vi "buntopenning.vi"() -> ()   [LabVIEW 2014, in "Panels.lvlib"]
uses:
  Panels.lvlib
  CSlibraries-extern/DimLVEvent/DimIndicators/DimIndicators.lvlib
  CSlibraries/UtilityLib/UtilityLib.lvlib
  CS_Core/CSSystem/CoreLib/CoreLib.lvlib
  CSlibraries/UtilityLib/UtilityLib.valueStatus.ctl
  CSlibraries-extern/DimLVEvent/LVDimInterface/LVDimInterface.lvlib
  Instance           1 20Saved   BuntoPenning .vi
  CSlibraries-extern/DimLVEvent/DimIndicators/DimIndicators.numericType.ctl
  CSlibraries-extern/DimLVEvent/DimIndicators/DimIndicators.numericArrayType.ctl
  CSlibraries-extern/DimLVEvent/DimIndicators/DimIndicators.anyType.ctl
panel:
  in  "SetFileLocation_Data":T1={"data"="NOLINK", "no link"=TRUE, "quality"=-1, "timeStamp"=0.0}
  in  "InjPenC":bool
  in  "InjPenB":bool
  in  "InjPenA":bool
  in  "InjPenBaseY":bool
  in  "InjPenBaseX":bool
  in  "InjPenDTBase1":bool
  in  "ELens8":bool
  in  "BOB5DefY":bool
  in  "BOB5DefX":bool
  in  "BOB4DefY":bool
  in  "BOB4DefX":bool
  in  "ELens7":bool
  in  "ELens6":bool
  in  "PulsedDT1":bool
  in  "PulsedDT2":bool
  in  "ELens8_SetData":T2={"data"=[0.0, 0.0, 0.0, 0.0], "no link"=FALSE, "quality"=0, "timeStamp"=3268667320.388}
  in  "SetFileLocation":path=path "\\\\intranet\\Files/projects/lebit/Data Exchange/data/buntopenningControl"
  in  "PulsedDT1_SetValueInfoData":T2={"data"=[-120.0, 120.0, -1.0], "no link"=FALSE, "quality"=0, "timeStamp"=3268667320.404}
  in  "PulsedDT1_SetData":T2={"data"=[0.0, 0.0, 0.0, 0.0], "no link"=FALSE, "quality"=0, "timeStamp"=3268667320.388}
  in  "PulsedDT1_MonData":T3={"data"=inf, "no link"=FALSE, "quality"=1, "timeStamp"=3268667320.373}
  in  "BOB4DefY_MonData":T3={"data"=inf, "no link"=FALSE, "quality"=1, "timeStamp"=3268667320.373}
  in  "ELens7_MonData":T3={"data"=inf, "no link"=FALSE, "quality"=1, "timeStamp"=3268667320.373}
  in  "BOB5DefX_MonData":T3={"data"=inf, "no link"=FALSE, "quality"=1, "timeStamp"=3268667320.373}
  in  "BOB5DefY_MonData":T3={"data"=inf, "no link"=FALSE, "quality"=1, "timeStamp"=3268667320.373}
  in  "ELens8_MonData":T3={"data"=inf, "no link"=TRUE, "quality"=-1, "timeStamp"=0.0}
  in  "InjPenDTBase1_MonData":T3={"data"=inf, "no link"=FALSE, "quality"=1, "timeStamp"=3268667320.373}
  in  "BOB4DefX_MonData":T3={"data"=inf, "no link"=FALSE, "quality"=1, "timeStamp"=3268667320.373}
  in  "ELens6_MonData":T3={"data"=inf, "no link"=FALSE, "quality"=1, "timeStamp"=3268667320.373}
  in  "BOB4Keithley_MonData":T3={"data"=inf, "no link"=FALSE, "quality"=1, "timeStamp"=3268667320.373}
  in  "PulsedDT2_MonData":T3={"data"=inf, "no link"=TRUE, "quality"=-1, "timeStamp"=0.0}
  in  "InjPenBaseY_MonData":T3={"data"=inf, "no link"=TRUE, "quality"=-1, "timeStamp"=0.0}
  in  "InjPenB_MonData":T3={"data"=inf, "no link"=FALSE, "quality"=1, "timeStamp"=3268667320.388}
  in  "InjPenBaseX_MonData":T3={"data"=inf, "no link"=TRUE, "quality"=-1, "timeStamp"=0.0}
  in  "InjPenA_MonData":T3={"data"=inf, "no link"=FALSE, "quality"=1, "timeStamp"=3268667320.388}
  in  "InjPenC_MonData":T3={"data"=inf, "no link"=FALSE, "quality"=1, "timeStamp"=3268667320.388}
  out "PulsedDT2_Mon":dbl=inf format="%.4f"
  out "InjPenC_Mon":dbl=inf format="%.4f"
  out "InjPenB_Mon":dbl=inf format="%.4f"
  out "InjPenA_Mon":dbl=inf format="%.4f"
  in  "PulsedDT2_SetValueInfoData":T2={"data"=[], "no link"=TRUE, "quality"=-1, "timeStamp"=0.0}
  in  "PulsedDT2_SetData":T2={"data"=[], "no link"=TRUE, "quality"=-1, "timeStamp"=0.0}
  in  "InjPenC_SetValueInfoData":T2={"data"=[0.0, 1500.0, -1.0], "no link"=FALSE, "quality"=0, "timeStamp"=3268667320.42}
  in  "InjPenBaseY_SetValueInfoData":T2={"data"=[], "no link"=TRUE, "quality"=-1, "timeStamp"=0.0}
  in  "InjPenBaseX_SetValueInfoData":T2={"data"=[], "no link"=TRUE, "quality"=-1, "timeStamp"=0.0}
  in  "InjPenB_SetValueInfoData":T2={"data"=[-400.0, 400.0, -1.0], "no link"=FALSE, "quality"=0, "timeStamp"=3268667320.42}
  in  "InjPenA_SetValueInfoData":T2={"data"=[-400.0, 400.0, -1.0], "no link"=FALSE, "quality"=0, "timeStamp"=3268667320.42}
  in  "InjPenC_SetData":T2={"data"=[0.0, 0.0, 0.0, 0.0], "no link"=FALSE, "quality"=0, "timeStamp"=3268667320.404}
  in  "InjPenBaseY_SetData":T2={"data"=[], "no link"=TRUE, "quality"=-1, "timeStamp"=0.0}
  in  "InjPenBaseX_SetData":T2={"data"=[], "no link"=TRUE, "quality"=-1, "timeStamp"=0.0}
  in  "InjPenB_SetData":T2={"data"=[0.0, 0.0, 0.0, 0.0], "no link"=FALSE, "quality"=0, "timeStamp"=3268667320.404}
  in  "InjPenA_SetData":T2={"data"=[0.0, 0.0, 0.0, 0.0], "no link"=FALSE, "quality"=0, "timeStamp"=3268667320.404}
  out "ELens7_Mon":dbl=inf format="%.4f"
  out "InjPenDTBase1_Mon":dbl=inf format="%.4f"
  out "ELens6_Mon":dbl=inf format="%.4f"
  out "ELens8_Mon":dbl=inf format="%.4f"
  out "InjPenBaseX_Mon":dbl=inf format="%.4f"
  out "PulsedDT1_Mon":dbl=inf format="%.4f"
  out "i ref out":refnum<vi>
  in  "Last Loaded File_Data":T1={"data"="NOLINK", "no link"=TRUE, "quality"=-1, "timeStamp"=0.0}
  out "FileUpToDate":bool=TRUE caption="Parameter Changed"
  in  "Close All Panels":bool
  in  "BOB4DefX_SetValueInfoData":T2={"data"=[], "no link"=TRUE, "quality"=-1, "timeStamp"=0.0}
  in  "BOB4DefY_SetValueInfoData":T2={"data"=[-400.0, 400.0, -1.0], "no link"=FALSE, "quality"=0, "timeStamp"=3268667320.42}
  in  "ELens7_SetValueInfoData":T2={"data"=[0.0, 5000.0, -1.0], "no link"=FALSE, "quality"=0, "timeStamp"=3268667320.42}
  in  "BOB5DefX_SetValueInfoData":T2={"data"=[-400.0, 400.0, -1.0], "no link"=FALSE, "quality"=0, "timeStamp"=3268667320.42}
  in  "BOB5DefY_SetValueInfoData":T2={"data"=[-400.0, 400.0, -1.0], "no link"=FALSE, "quality"=0, "timeStamp"=3268667320.42}
  in  "ELens8_SetValueInfoData":T2={"data"=[], "no link"=TRUE, "quality"=-1, "timeStamp"=0.0}
  in  "InjPenDTBase1_SetValueInfoData":T2={"data"=[0.0, 3000.0, -1.0], "no link"=FALSE, "quality"=0, "timeStamp"=3268667320.42}
  in  "ELens6_SetValueInfoData":T2={"data"=[0.0, 5000.0, -1.0], "no link"=FALSE, "quality"=0, "timeStamp"=3268667320.404}
  in  "InjPenDTBase1_SetData":T2={"data"=[0.0, 0.0, 0.0, 0.0], "no link"=FALSE, "quality"=0, "timeStamp"=3268667320.388}
  in  "BOB5DefY_SetData":T2={"data"=[0.0, 0.0, 0.0, 0.0], "no link"=FALSE, "quality"=0, "timeStamp"=3268667320.388}
  in  "BOB5DefX_SetData":T2={"data"=[0.0, 0.0, 0.0, 0.0], "no link"=FALSE, "quality"=0, "timeStamp"=3268667320.388}
  in  "ELens7_SetData":T2={"data"=[0.0, 0.0, 0.0, 0.0], "no link"=FALSE, "quality"=0, "timeStamp"=3268667320.388}
  in  "BOB4DefY_SetData":T2={"data"=[0.0, 0.0, 0.0, 0.0], "no link"=FALSE, "quality"=0, "timeStamp"=3268667320.388}
  in  "BOB4DefX_SetData":T2={"data"=[0.0, 0.0, 0.0, 0.0], "no link"=FALSE, "quality"=0, "timeStamp"=3268667320.388}
  in  "ELens6_SetData":T2={"data"=[0.0, 0.0, 0.0, 0.0], "no link"=FALSE, "quality"=0, "timeStamp"=3268667320.388}
  out "Last Loaded File":string
  out "BOB5DefY_Mon":dbl=inf format="%.4f"
  out "InjPenBaseY_Mon":dbl=inf format="%.4f"
  out "BOB4DefY_Mon":dbl=inf format="%.4f"
  out "BOB5DefX_Mon":dbl=inf format="%.4f"
  out "BOB4DefX_Mon":dbl=inf format="%.4f"
  # "Parameter changed, data file is no longer up-to-date."
  # "Values in italic don't have a real monitor"
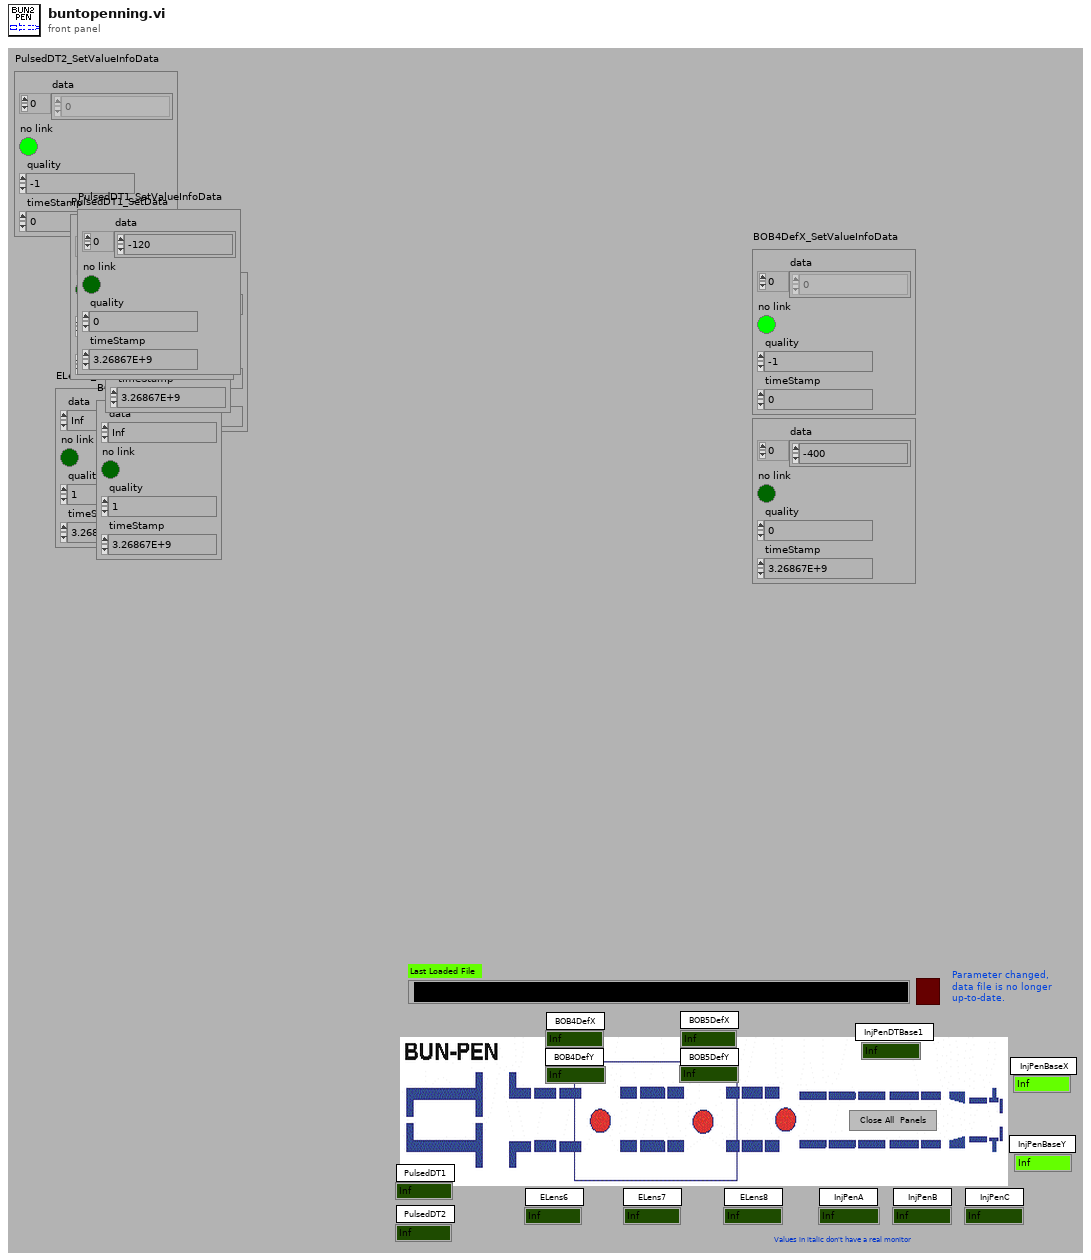
[diagram p1: front panel]
types:
  T1 = typedef "DimIndicators.lvlib/DimIndicators.anyType.ctl" = cluster{"data":string, "no link":bool, "quality":i32, "timeStamp":dbl}
  T2 = typedef "DimIndicators.lvlib/DimIndicators.numericArrayType.ctl" = cluster{"data":dbl[], "no link":bool, "quality":i32, "timeStamp":dbl}
  T3 = typedef "DimIndicators.lvlib/DimIndicators.numericType.ctl" = cluster{"data":dbl, "no link":bool, "quality":i32, "timeStamp":dbl}
  T4 = typedef "UtilityLib.lvlib/UtilityLib.valueStatus.ctl" = enum16{"no info available", "stand by/off", "on", "warning", "alarm/malfunction", "not implemented", "user action required", "important information", "system default", "control default", "indicator default", "button default"}
  T5 = cluster{"data":string, "no link":bool, "quality":i32, "timeStamp":dbl}
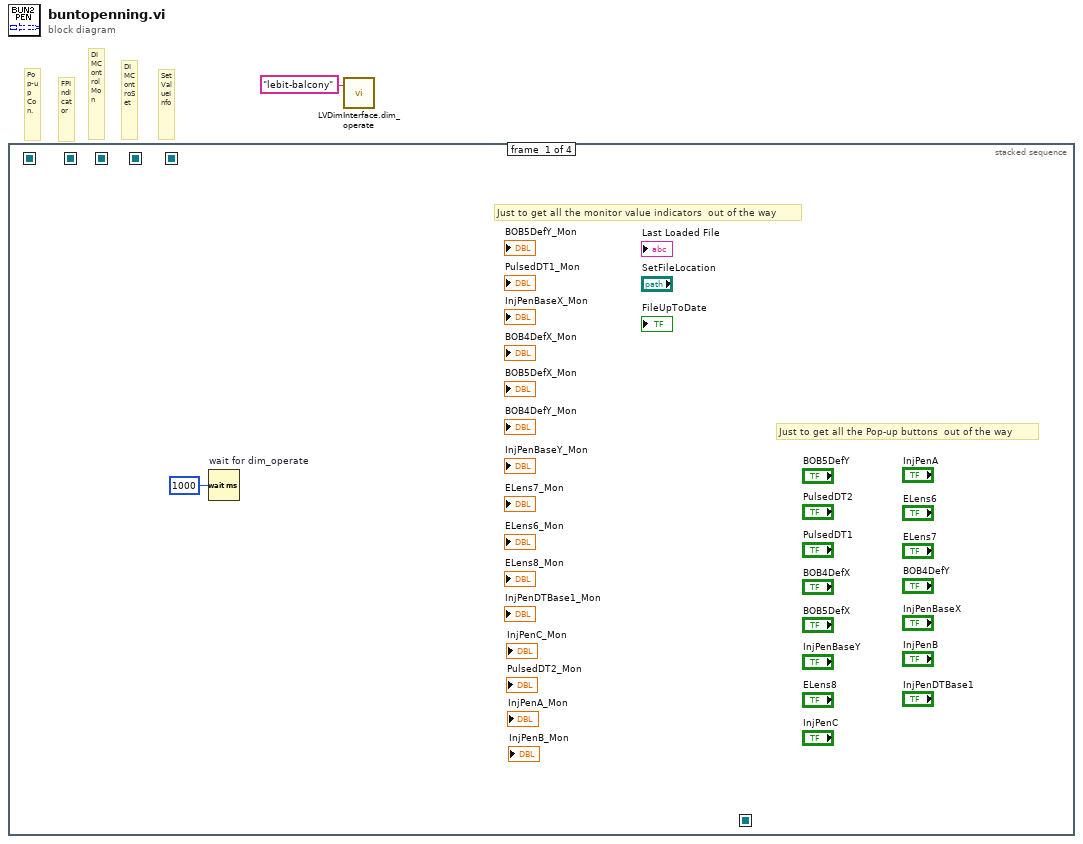
[diagram p0: block diagram]
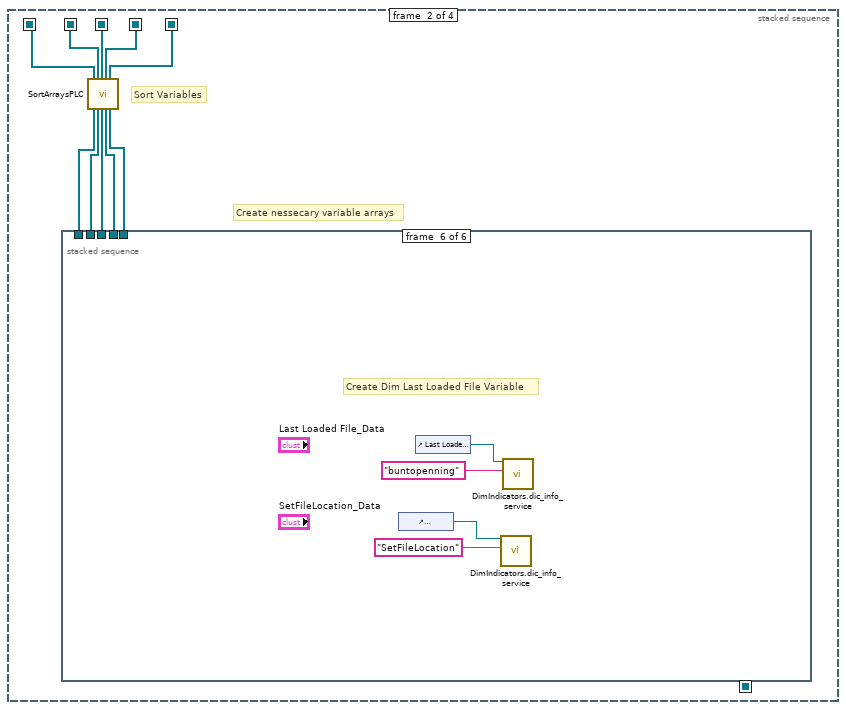
[diagram p2: hidden frame]
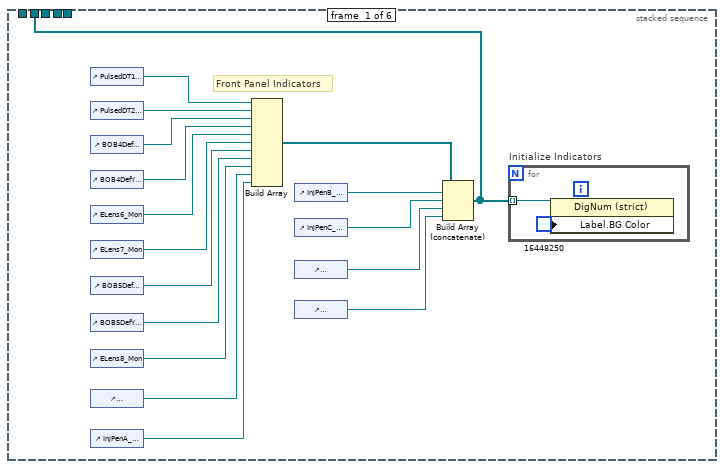
[diagram p3: hidden frame]
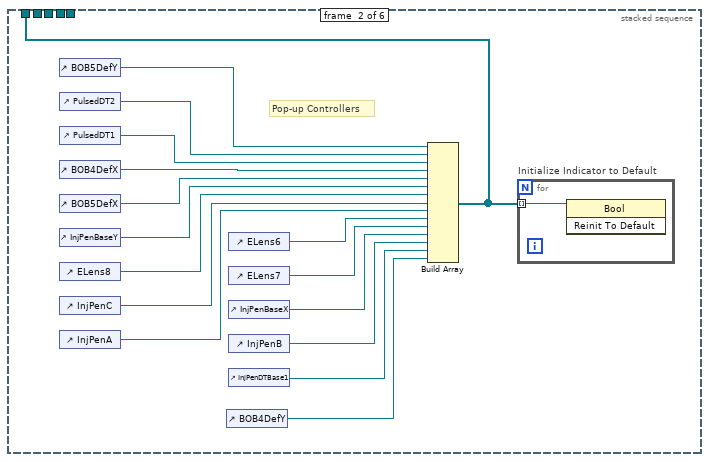
[diagram p4: hidden frame]
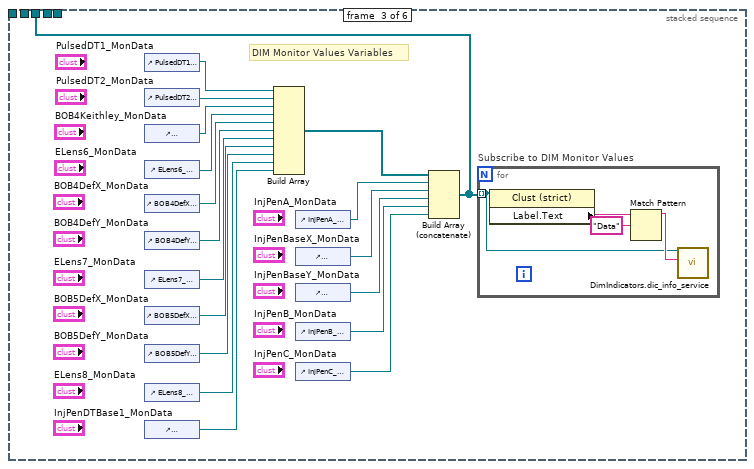
[diagram p5: hidden frame]
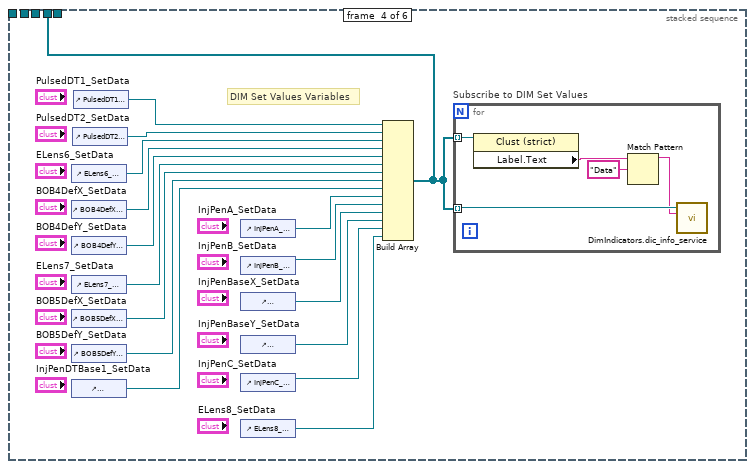
[diagram p6: hidden frame]
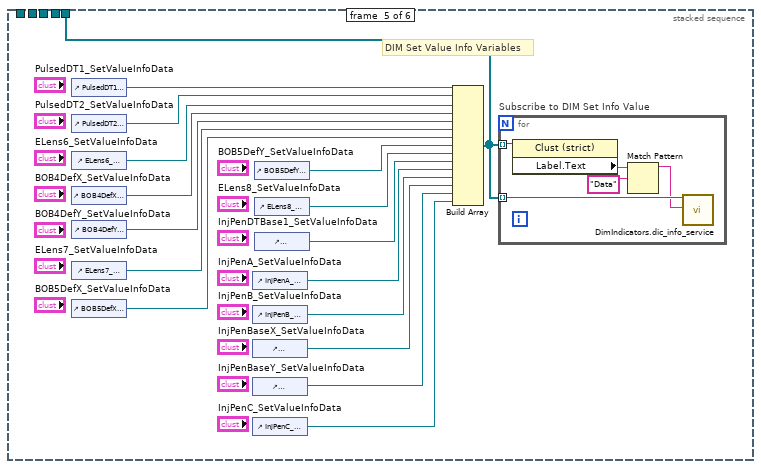
[diagram p7: hidden frame]
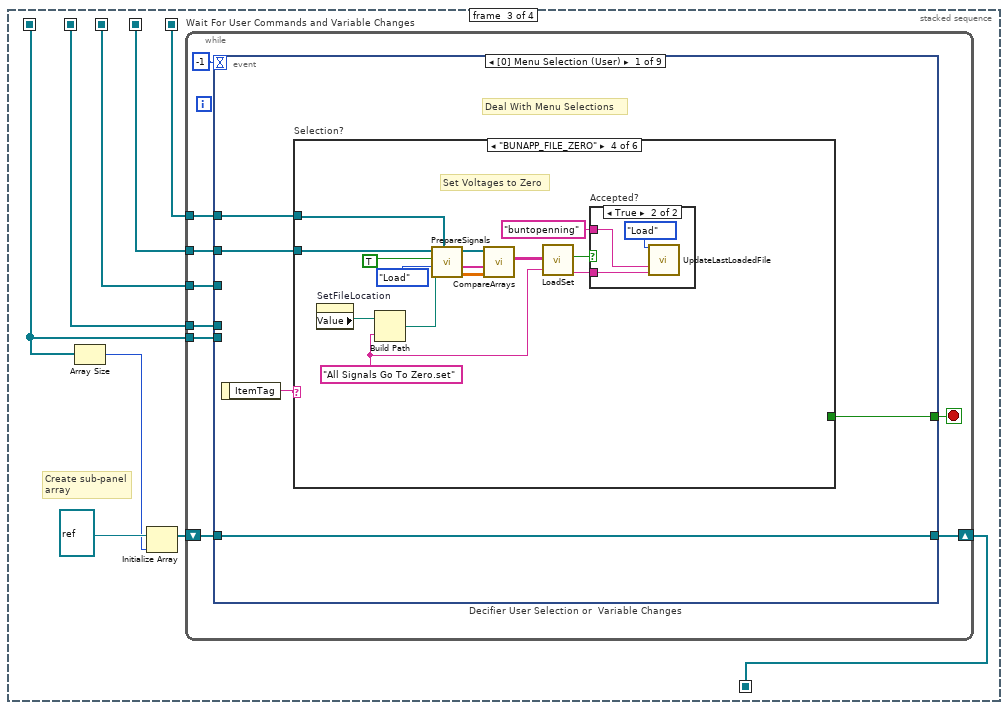
[diagram p8: hidden frame]
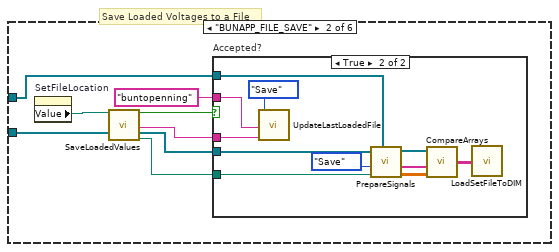
[diagram p10: hidden frame]
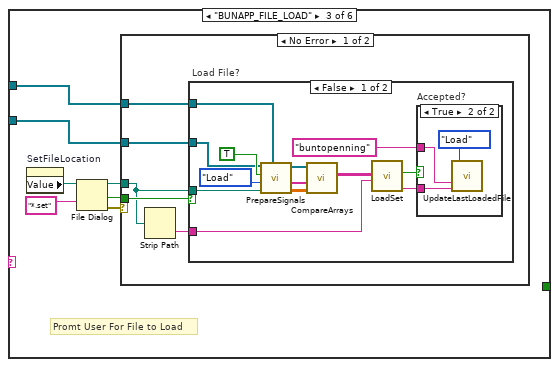
[diagram p12: hidden frame]
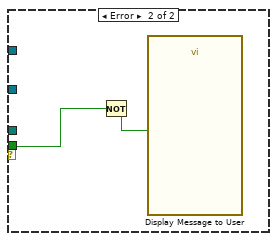
[diagram p15: hidden frame]
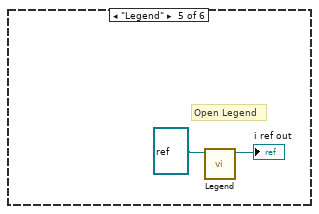
[diagram p17: hidden frame]
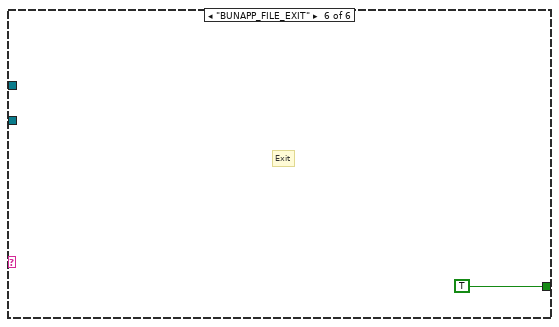
[diagram p18: hidden frame]
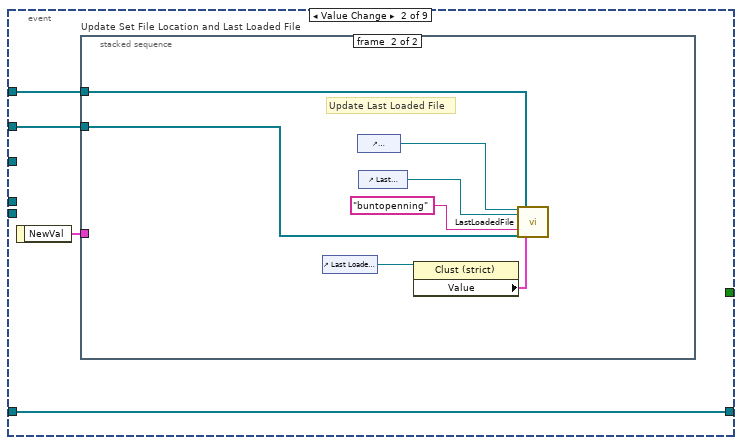
[diagram p19: hidden frame]
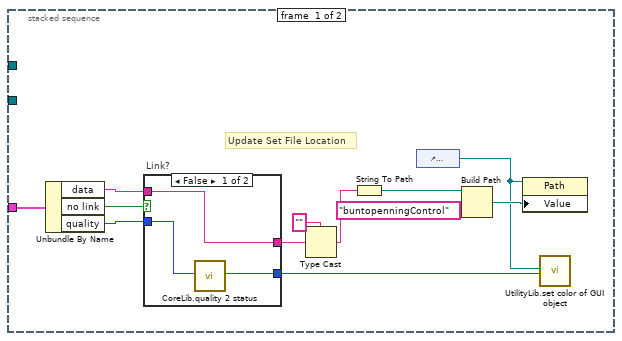
[diagram p20: hidden frame]
diagram:
  # "Pop-up Con."
  # "SetValueInfo"
  # "DIMControSet"
  # "DIMControlMon"
  # "FPIndicator"
  n1 = stacked-sequence {
    seq-local: [_ w8 _ _] -> [_ _ w119 _]
    seq-local: [_ w10 _ _] -> [_ _ w117 w318]
    seq-local: [_ _ w122 _] -> [_ _ _ w317]
    seq-local: [_ w11 _ _] -> [_ _ w121 w316]
    seq-local: [_ w12 _ _] -> [_ _ w118 w315]
    seq-local: [_ w9 _ _] -> [_ _ w120 _]
    frame #0 {
      # "Just to get all the Pop-up buttons  out of the way"
      # "Just to get all the monitor value indicators  out of the way"
      n2 = Wait (ms) "wait for dim_operate"(milliseconds to wait=u32 1000) -> ()  [unwired: 1 out]
    }
    frame #1 {
      # "Create nessecary variable arrays"
      # "Sort Variables"
      n3 = stacked-sequence {
        tunnel: [w13 _ _ _ _ _] -> w7
        tunnel: [_ w32 _ _ _ _] -> w6
        tunnel: [_ _ w49 _ _ _] -> w5
        tunnel: [_ _ _ w71 _ _] -> w4
        tunnel: [_ _ _ _ w92 _] -> w3
        frame #0 {
          # "Front Panel Indicators"
          n4 = control-ref of="PulsedDT1_Mon"() -> (w29:refnum<vi>)
          n5 = control-ref of="PulsedDT2_Mon"() -> (w25:refnum<vi>)
          n6 = control-ref of="BOB4DefX_Mon"() -> (w28:refnum<vi>)
          n7 = control-ref of="BOB4DefY_Mon"() -> (w24:refnum<vi>)
          n8 = control-ref of="ELens6_Mon"() -> (w23:refnum<vi>)
          n9 = control-ref of="ELens7_Mon"() -> (w22:refnum<vi>)
          n10 = control-ref of="BOB5DefX_Mon"() -> (w21:refnum<vi>)
          n11 = control-ref of="BOB5DefY_Mon"() -> (w20:refnum<vi>)
          n12 = control-ref of="ELens8_Mon"() -> (w19:refnum<vi>)
          n13 = control-ref of="InjPenDTBase1_Mon"() -> (w18:refnum<vi>)
          n14 = control-ref of="InjPenA_Mon"() -> (w17:refnum<vi>)
          n15 = Build Array(w29, w25, w28, w24, w23, w22, w21, w20, w19, w18, w17) -> (w27:refnum<vi>[])
          n16 = control-ref of="InjPenB_Mon"() -> (w16:refnum<vi>)
          n17 = control-ref of="InjPenC_Mon"() -> (w26:refnum<vi>)
          n18 = control-ref of="InjPenBaseX_Mon"() -> (w15:refnum<vi>)
          n19 = control-ref of="InjPenBaseY_Mon"() -> (w14:refnum<vi>)
          n20 = Build Array (concatenate)(w27, w16, w26, w15, w14) -> (w13:refnum<vi>[])
          n21 = for "Initialize Indicators" {
            tunnel: w13 -> [w31] mode=indexing
            n22 = property class="DigNum (strict)"(reference=w31, "Label.BG Color"=u32 16448250 ("Color Box")) -> ()  [unwired: 1 in, 2 out]
          }
        }
        frame #1 {
          # "Pop-up Controllers"
          n23 = control-ref of="BOB5DefY"() -> (w47:refnum<vi>)
          n24 = control-ref of="PulsedDT2"() -> (w46:refnum<vi>)
          n25 = control-ref of="PulsedDT1"() -> (w45:refnum<vi>)
          n26 = control-ref of="BOB4DefX"() -> (w44:refnum<vi>)
          n27 = control-ref of="BOB5DefX"() -> (w43:refnum<vi>)
          n28 = control-ref of="InjPenBaseY"() -> (w42:refnum<vi>)
          n29 = control-ref of="ELens8"() -> (w41:refnum<vi>)
          n30 = control-ref of="InjPenC"() -> (w40:refnum<vi>)
          n31 = control-ref of="InjPenA"() -> (w39:refnum<vi>)
          n32 = control-ref of="BOB4DefY"() -> (w33:refnum<vi>)
          n33 = control-ref of="ELens6"() -> (w38:refnum<vi>)
          n34 = control-ref of="ELens7"() -> (w37:refnum<vi>)
          n35 = control-ref of="InjPenBaseX"() -> (w36:refnum<vi>)
          n36 = control-ref of="InjPenB"() -> (w35:refnum<vi>)
          n37 = control-ref of="InjPenDTBase1"() -> (w34:refnum<vi>)
          n38 = Build Array(w47, w46, w45, w44, w43, w42, w41, w40, w39, w38, w37, w36, w35, w34, w33) -> (w32:refnum<vi>[])
          n39 = for "Initialize Indicator to Default" {
            tunnel: w32 -> [w48] mode=indexing
            n40 = invoke class="Bool" method="Reinit To Default"(reference=w48) -> ()  [unwired: 2 in, 3 out]
          }
        }
        frame #2 {
          # "DIM Monitor Values Variables"
          n41 = control-ref of="PulsedDT1_MonData"() -> (w50:refnum<vi>)
          n42 = control-ref of="PulsedDT2_MonData"() -> (w51:refnum<vi>)
          n43 = control-ref of="BOB4Keithley_MonData"() -> (w56:refnum<vi>)
          n44 = control-ref of="ELens6_MonData"() -> (w60:refnum<vi>)
          n45 = control-ref of="BOB4DefX_MonData"() -> (w59:refnum<vi>)
          n46 = control-ref of="BOB4DefY_MonData"() -> (w66:refnum<vi>)
          n47 = control-ref of="ELens7_MonData"() -> (w65:refnum<vi>)
          n48 = control-ref of="BOB5DefX_MonData"() -> (w64:refnum<vi>)
          n49 = control-ref of="BOB5DefY_MonData"() -> (w63:refnum<vi>)
          n50 = control-ref of="ELens8_MonData"() -> (w62:refnum<vi>)
          n51 = control-ref of="InjPenDTBase1_MonData"() -> (w61:refnum<vi>)
          n52 = Build Array(w50, w51, w56, w60, w59, w66, w65, w64, w63, w62, w61) -> (w53:refnum<vi>[])
          n53 = control-ref of="InjPenA_MonData"() -> (w58:refnum<vi>)
          n54 = control-ref of="InjPenBaseX_MonData"() -> (w57:refnum<vi>)
          n55 = control-ref of="InjPenBaseY_MonData"() -> (w55:refnum<vi>)
          n56 = control-ref of="InjPenB_MonData"() -> (w54:refnum<vi>)
          n57 = control-ref of="InjPenC_MonData"() -> (w52:refnum<vi>)
          n58 = Build Array (concatenate)(w53, w58, w57, w55, w54, w52) -> (w49:refnum<vi>[])
          n59 = for "Subscribe to DIM Monitor Values" {
            tunnel: w49 -> [w67] mode=indexing
            n60 = property class="Clust (strict)"(reference=w67) -> ("Label.Text"=w69:string)  [unwired: 1 in, 2 out]
            n61 = Match Pattern(string=w69, regular expression="Data") -> (before substring=w68:string)  [unwired: 1 in, 3 out]
            n62 = call "DimIndicators.dic_info_service.vi"("controlRef"=w67, "serviceName"=w68) -> ()  [unwired: 16 in, 2 out]
          }
        }
        frame #3 {
          # "DIM Set Values Variables"
          n63 = control-ref of="ELens6_SetData"() -> (w86:refnum<vi>)
          n64 = control-ref of="BOB4DefX_SetData"() -> (w85:refnum<vi>)
          n65 = control-ref of="BOB4DefY_SetData"() -> (w84:refnum<vi>)
          n66 = control-ref of="ELens7_SetData"() -> (w83:refnum<vi>)
          n67 = control-ref of="BOB5DefX_SetData"() -> (w82:refnum<vi>)
          n68 = control-ref of="BOB5DefY_SetData"() -> (w81:refnum<vi>)
          n69 = control-ref of="InjPenDTBase1_SetData"() -> (w80:refnum<vi>)
          n70 = control-ref of="PulsedDT2_SetData"() -> (w75:refnum<vi>)
          n71 = control-ref of="PulsedDT1_SetData"() -> (w73:refnum<vi>)
          n72 = control-ref of="InjPenA_SetData"() -> (w74:refnum<vi>)
          n73 = control-ref of="InjPenB_SetData"() -> (w79:refnum<vi>)
          n74 = control-ref of="InjPenBaseX_SetData"() -> (w78:refnum<vi>)
          n75 = control-ref of="InjPenBaseY_SetData"() -> (w77:refnum<vi>)
          n76 = control-ref of="InjPenC_SetData"() -> (w76:refnum<vi>)
          n77 = control-ref of="ELens8_SetData"() -> (w72:refnum<vi>)
          n78 = Build Array(w73, w75, w86, w85, w84, w83, w82, w81, w80, w74, w79, w78, w77, w76, w72) -> (w71:refnum<vi>[])
          n79 = for "Subscribe to DIM Set Values" {
            tunnel: w71 -> [w87] mode=indexing
            tunnel: w71 -> [w91] mode=indexing
            n80 = property class="Clust (strict)"(reference=w87) -> ("Label.Text"=w90:string)  [unwired: 1 in, 2 out]
            n81 = Match Pattern(string=w90, regular expression="Data") -> (before substring=w88:string)  [unwired: 1 in, 3 out]
            n82 = call "DimIndicators.dic_info_service.vi"("controlRef"=w91, "serviceName"=w88) -> ()  [unwired: 16 in, 2 out]
          }
        }
        frame #4 {
          # "DIM Set Value Info Variables"
          n83 = control-ref of="PulsedDT1_SetValueInfoData"() -> (w93:refnum<vi>)
          n84 = control-ref of="PulsedDT2_SetValueInfoData"() -> (w94:refnum<vi>)
          n85 = control-ref of="ELens6_SetValueInfoData"() -> (w107:refnum<vi>)
          n86 = control-ref of="BOB4DefX_SetValueInfoData"() -> (w106:refnum<vi>)
          n87 = control-ref of="BOB4DefY_SetValueInfoData"() -> (w105:refnum<vi>)
          n88 = control-ref of="ELens7_SetValueInfoData"() -> (w104:refnum<vi>)
          n89 = control-ref of="BOB5DefX_SetValueInfoData"() -> (w103:refnum<vi>)
          n90 = control-ref of="InjPenA_SetValueInfoData"() -> (w99:refnum<vi>)
          n91 = control-ref of="InjPenB_SetValueInfoData"() -> (w98:refnum<vi>)
          n92 = control-ref of="InjPenBaseX_SetValueInfoData"() -> (w97:refnum<vi>)
          n93 = control-ref of="InjPenBaseY_SetValueInfoData"() -> (w96:refnum<vi>)
          n94 = control-ref of="InjPenC_SetValueInfoData"() -> (w95:refnum<vi>)
          n95 = control-ref of="BOB5DefY_SetValueInfoData"() -> (w102:refnum<vi>)
          n96 = control-ref of="ELens8_SetValueInfoData"() -> (w101:refnum<vi>)
          n97 = control-ref of="InjPenDTBase1_SetValueInfoData"() -> (w100:refnum<vi>)
          n98 = Build Array(w93, w94, w107, w106, w105, w104, w103, w102, w101, w100, w99, w98, w97, w96, w95) -> (w92:refnum<vi>[])
          n99 = for "Subscribe to DIM Set Info Value" {
            tunnel: w92 -> [w108] mode=indexing
            tunnel: w92 -> [w112] mode=indexing
            n100 = property class="Clust (strict)"(reference=w108) -> ("Label.Text"=w111:string)  [unwired: 1 in, 2 out]
            n101 = Match Pattern(string=w111, regular expression="Data") -> (before substring=w109:string)  [unwired: 1 in, 3 out]
            n102 = call "DimIndicators.dic_info_service.vi"("controlRef"=w112, "serviceName"=w109) -> ()  [unwired: 16 in, 2 out]
          }
        }
        frame #5 {
          # "Create Dim Last Loaded File Variable"
          n103 = control-ref of="SetFileLocation_Data"() -> (w116:refnum<vi>)
          n104 = control-ref of="Last Loaded File_Data"() -> (w114:refnum<vi>)
          n105 = call "DimIndicators.dic_info_service.vi"("controlRef"=w116, "serviceName"="SetFileLocation" ("string")) -> ()  [unwired: 16 in, 2 out]
          n106 = call "DimIndicators.dic_info_service.vi"("controlRef"=w114, "serviceName"="buntopenning" ("string")) -> ()  [unwired: 16 in, 2 out]
        }
      }
      n107 = call "SortArraysPLC.vi"("Pop-up Con."=w6, "FPIndicator in"=w7, "DIMControlMon"=w5, "DIMControSet"=w4, "SetValueInfo"=w3) -> ("Pop-up Con. out"=w9:refnum<vi>[], "FPIndicator out"=w8:refnum<vi>[], "DIMControlMon out"=w10:refnum<vi>[], "DIMControSet out"=w11:refnum<vi>[], "SetValueInfo out"=w12:refnum<vi>[])  [unwired: 18 in]
    }
    frame #2 {
      # "Create sub-panel\narray"
      n108 = Array Size(array=w120) -> (size(s)=w123:i32)
      n109 = Initialize Array(refnum<vi> refnum ("vi reference"), w123) -> (w125:refnum<vi>[])
      n110 = while "Wait For User Commands and Variable Changes" {
        shift-right: [w132] -> w122
        shift-left: w125 -> [w133]
        tunnel: w121 -> [w130]
        tunnel: w120 -> [w129]
        tunnel: w119 -> [w128]
        tunnel: w118 -> [w127]
        tunnel: w117 -> [w126]
        stop <- w134 stop-if-true
        n111 = event "Decifier User Selection or  Variable Changes" shown="[0] Menu Selection (User)" {
          selector: _ -> [_ _ _ _ _ _ _ _ _]
          dyn-events: _ -> [_ _ _ _ _ _ _ _ _]
          timeout: -1 -> [_ _ _ _ _ _ _ _ _]
          tunnel: [w137 _ _ _ _ _ _ _ TRUE ("stop")] -> w134
          tunnel: w133 -> [w139 w211 w243 w248 w255 w276 w283 w289 w290]
          tunnel: [w139 w211 w243 w248 w255 w274 w281 w289 _] -> w132
          tunnel: w130 -> [w136 w210 w238 w247 _ _ _ _ w292]
          tunnel: w129 -> [_ _ _ _ _ w269 _ _ _]
          tunnel: w128 -> [_ _ _ _ w251 _ _ _ _]
          tunnel: w127 -> [w135 w209 w237 _ _ _ _ _ w293]
          tunnel: w126 -> [_ _ _ _ w253 _ _ _ w291]
          event Menu Selection (User) {
            # "Deal With Menu Selections"
            n112 = event-data() -> ("ItemTag"=w138:string)  [unwired: 1 in]
            n113 = case "Selection?" shown="\"BUNAPP_FILE_ZERO\"" w138 {
              tunnel: [_ _ _ _ _ TRUE ("stop")] -> w137
              tunnel: w135 -> [_ w140 w160 w190 _ _]
              tunnel: w136 -> [_ w141 w159 w189 _ _]
              frame "False", Default {
              }
              frame "BUNAPP_FILE_SAVE" {
                # "Save Loaded Voltages to a File"
                n114 = property on="SetFileLocation" class="Path"() -> ("Value"=w145:path)  [unwired: 2 in, 2 out]
                n115 = call "SaveLoadedValues.vi"("Panel Location?"=w145, "DIMControlSet in"=w141) -> ("File Saved?"=w146:bool, "File Name"=w144:string, "DIMControlSet out"=w142:refnum<vi>[], "Path"=w143:path)  [unwired: 14 in]
                n116 = case "Accepted?" shown="True" w146 {
                  tunnel: w144 -> [_ w156]
                  tunnel: "buntopenning" ("string") -> [_ w158]
                  tunnel: w142 -> [_ w157]
                  tunnel: w143 -> [_ w155]
                  tunnel: w140 -> [_ w149]
                  frame False {
                  }
                  frame True {
                    n117 = call "UpdateLastLoadedFile.vi"("LoadOrSave"=enum16{"Load", "Save"}."Save", "GUIName"=w158, "FileNameIn"=w156) -> ()  [unwired: 13 in]
                    n118 = call "PrepareSignals.vi"("SetValueInfo in"=w149, "setfile path"=w155, "Enum"=enum16{"Save", "Load"}."Save", "DIMControSet in"=w157) -> ("indexed loaded Array"=w153:dbl[][], "Name Array"=w154:string[], "DIMControSet out"=w152:refnum<vi>[])  [unwired: 5 in]
                    n119 = call "CompareArrays.vi"("indexed loaded Array"=w153, "Name Array"=w154, "DIMControSet"=w152) -> ("Table for loading values"=w151:string[][])  [unwired: 4 in]
                    n120 = call "LoadSetFileToDIM.vi"("output array"=w151) -> ()  [unwired: 2 in]
                  }
                }
              }
              frame "BUNAPP_FILE_LOAD" {
                # "Promt User For File to Load"
                n121 = property on="SetFileLocation" class="Path"() -> ("Value"=w162:path)  [unwired: 2 in, 2 out]
                n122 = File Dialog(6:"*.set" ("pattern (all files)"), 11:w162) -> (0:w161:errorcluster, 1:w165:bool, 3:w163:path)  [unwired: 5 in, 1 out]
                n123 = case shown="No Error" w161 {
                  tunnel: w165 -> [w170 w187]
                  tunnel: w163 -> [w168 _]
                  tunnel: w160 -> [w167 _]
                  tunnel: w159 -> [w166 _]
                  frame No Error {
                    n124 = Strip Path(path=w168) -> (name=w169:string)  [unwired: 1 out]
                    n125 = case "Load File?" shown="False" w170 {
                      tunnel: w169 -> [w178 _]
                      tunnel: w168 -> [w179 _]
                      tunnel: w167 -> [w172 _]
                      tunnel: w166 -> [w171 _]
                      frame False {
                        n126 = call "PrepareSignals.vi"("SetValueInfo in"=w172, "setfile path"=w179, "Enum"=enum16{"Save", "Load"}."Load", "Display Message to \nUser"=TRUE ("Display Message to \nUser"), "DIMControSet in"=w171) -> ("indexed loaded Array"=w182:dbl[][], "Name Array"=w181:string[], "DIMControSet out"=w183:refnum<vi>[])  [unwired: 4 in]
                        n127 = call "CompareArrays.vi"("indexed loaded Array"=w182, "Name Array"=w181, "DIMControSet"=w183) -> ("Table for loading values"=w180:string[][])  [unwired: 4 in]
                        n128 = call "LoadSet.vi"("File Name In"=w178, "output array"=w180) -> ("File Name out"=w177:string, "Accepted"=w176:bool)  [unwired: 8 in]
                        n129 = case "Accepted?" shown="True" w176 {
                          tunnel: w177 -> [_ w186]
                          tunnel: "buntopenning" ("string") -> [_ w185]
                          frame False {
                          }
                          frame True {
                            n130 = call "UpdateLastLoadedFile.vi"("LoadOrSave"=enum16{"Load", "Save"}."Load", "GUIName"=w185, "FileNameIn"=w186) -> ()  [unwired: 13 in]
                          }
                        }
                      }
                      frame True {
                      }
                    }
                  }
                  frame Error {
                    n131 = Not(x=w187) -> (.not. x?=w188:bool)
                    n132 = call "Display Message to User"("Enable"=w188) -> ()  [unwired: 9 in, 2 out]
                  }
                }
              }
              frame "BUNAPP_FILE_ZERO" {
                w194 = "All Signals Go To Zero.set" ("File Name")
                # "Set Voltages to Zero"
                n133 = property on="SetFileLocation" class="Path"() -> ("Value"=w192:path)  [unwired: 2 in, 2 out]
                n134 = Build Path(base path=w192, name or relative path=w194) -> (appended path=w193:path)
                n135 = call "PrepareSignals.vi"("SetValueInfo in"=w190, "setfile path"=w193, "Enum"=enum16{"Save", "Load"}."Load", "Display Message to \nUser"=TRUE ("Display Message to \nUser"), "DIMControSet in"=w189) -> ("indexed loaded Array"=w201:dbl[][], "Name Array"=w200:string[], "DIMControSet out"=w202:refnum<vi>[])  [unwired: 4 in]
                n136 = call "CompareArrays.vi"("indexed loaded Array"=w201, "Name Array"=w200, "DIMControSet"=w202) -> ("Table for loading values"=w199:string[][])  [unwired: 4 in]
                n137 = call "LoadSet.vi"("File Name In"=w194, "output array"=w199) -> ("File Name out"=w197:string, "Accepted"=w198:bool)  [unwired: 8 in]
                n138 = case "Accepted?" shown="True" w198 {
                  tunnel: w197 -> [_ w205]
                  tunnel: "buntopenning" ("string") -> [_ w204]
                  frame False {
                  }
                  frame True {
                    n139 = call "UpdateLastLoadedFile.vi"("LoadOrSave"=enum16{"Load", "Save"}."Load", "GUIName"=w204, "FileNameIn"=w205) -> ()  [unwired: 13 in]
                  }
                }
              }
              frame "Legend" {
                # "Open Legend"
                n140 = call "Legend.vi"("i ref in"=refnum<vi> refnum) -> ("i ref out"=→"i ref out":refnum<vi>)  [unwired: 10 in]
              }
              frame "BUNAPP_FILE_EXIT" {
                # "Exit"
              }
            }
          }
          event Value Change {
            n141 = event-data() -> ("NewVal"=w212:T1)  [unwired: 1 in]
            n142 = stacked-sequence "Update Set File Location and Last Loaded File" {
              tunnel: w210 -> [_ w234]
              tunnel: w212 -> [w214 _]
              tunnel: w209 -> [_ w230]
              frame #0 {
                # "Update Set File Location"
                n143 = Unbundle By Name(w214) -> ("data"=w223:string, "no link"=w222:bool, "quality"=w221:i32)
                n144 = case "Link?" shown="False" w222 {
                  tunnel: w221 -> [w227 _]
                  tunnel: [w226 UtilityLib.valueStatus."no info available" ("valueStatus")] -> w224
                  tunnel: w223 -> [w225 _]
                  tunnel: [w225 w228] -> w219
                  frame False {
                    n145 = call "CoreLib.quality 2 status.vi"("quality"=w227) -> ("valueStatus"=w226:T4)  [unwired: 18 in]
                  }
                  frame True {
                    n146 = call "EmptyString.vi"() -> ("String"=w228:string)
                  }
                }
                n147 = Type Cast(type="" ("regular expression"), x=w219) -> (*(type *) &x=w218:string)
                n148 = String To Path(string=w218) -> (path=w215:path)
                n149 = control-ref of="SetFileLocation"() -> (w213:refnum<vi>)
                n150 = Build Path(base path=w215, name or relative path="buntopenningControl") -> (appended path=w216:path)
                n151 = property class="Path"(reference=w213, "Value"=w216) -> ()  [unwired: 1 in, 2 out]
                n152 = call "UtilityLib.set color of GUI object.vi"("GUI object Ref"=w213, "valueStatus"=w224) -> ()  [unwired: 17 in, 1 out]
              }
              frame #1 {
                # "Update Last Loaded File"
                n153 = control-ref of="Last Loaded File_Data"() -> (w231:refnum<vi>)
                n154 = control-ref of="SetFileLocation"() -> (w236:refnum<vi>)
                n155 = control-ref of="Last Loaded File"() -> (w235:refnum<vi>)
                n156 = property class="Clust (strict)"(reference=w231) -> ("Value"=w233:T5)  [unwired: 1 in, 2 out]
                n157 = call "LastLoadedFile.vi"("SetFileLocation"=w236, "Last Loaded File"=w235, "GUIName"="buntopenning", "DIMControSet in"=w234, "SetValueInfo in"=w230, "NewVal"=w233) -> ()  [unwired: 14 in]
              }
            }
          }
          event Value Change {
            # "Update Last Loaded File"
            n158 = event-data() -> ("NewVal"=w242:T1)  [unwired: 1 in]
            n159 = control-ref of="SetFileLocation"() -> (w239:refnum<vi>)
            n160 = control-ref of="Last Loaded File"() -> (w240:refnum<vi>)
            n161 = call "LastLoadedFile.vi"("SetFileLocation"=w239, "Last Loaded File"=w240, "GUIName"="bun", "DIMControSet in"=w238, "SetValueInfo in"=w237, "NewVal"=w242) -> ()  [unwired: 14 in]
          }
          event Value Change {
            n162 = event-data() -> ("CtlRef"=w246:refnum<vi>)  [unwired: 1 in, 5 out]
            n163 = property on="FileUpToDate" class="Bool (strict)"() -> ("Value"=w244:bool)  [unwired: 2 in, 2 out]
            n164 = call "FileUpToDate.vi"("FileUpToDate in"=w244, "DIMControSet out"=w247, "CtlRef"=w246) -> ("FileUpToDate out"=w245:bool)  [unwired: 16 in]
            n165 = property on="FileUpToDate" class="Bool (strict)"("Value"=w245) -> ()  [unwired: 2 in, 2 out]
          }
          event Value Change {
            # "Find Monitor Value Index"
            # "Updating a Monitor Value"
            n166 = event-data() -> ("CtlRef"=w252:refnum<vi>, "NewVal"=w256:T3)  [unwired: 1 in, 4 out]
            n167 = Search 1D Array(1D array=w253, element=w252) -> (index of element=w254:i32)  [unwired: 1 in]
            n168 = Index Array(array=w251, index=w254) -> (element=w250:refnum<vi>)
            n169 = Not A Number/Path/Refnum?(number/path/refnum=w250) -> (NaN/Path/Refnum?=w249:bool)
            n170 = case "Indicator exists?" shown="False" w249 {
              tunnel: w256 -> [_ w263]
              tunnel: w250 -> [_ w257]
              frame True {
              }
              frame False {
                n171 = Unbundle By Name(w263) -> ("data"=w259:dbl, "no link"=w260:bool, "quality"=w262:i32)
                n172 = case shown="False" w260 {
                  tunnel: w262 -> [w266 _]
                  tunnel: [w265 UtilityLib.valueStatus."no info available" ("valueStatus")] -> w261
                  tunnel: w259 -> [w264 _]
                  tunnel: [w264 inf] -> w258
                  frame False {
                    n173 = call "CoreLib.quality 2 status.vi"("quality"=w266) -> ("valueStatus"=w265:T4)  [unwired: 18 in]
                  }
                  frame True {
                  }
                }
                n174 = property class="DigNum (strict)"(reference=w257, "Value"=w258) -> ()  [unwired: 1 in, 2 out]
                n175 = call "TextColor.vi"("valueStatus"=w261, "reference"=w257) -> ()  [unwired: 10 in]
              }
            }
          }
          event "PulsedDT2", "PulsedDT1", "ELens6", "ELens7", "BOB4DefX", "BOB4DefY", "BOB5DefX", "ELens8", "InjPenDTBase1", "InjPenBaseX", "InjPenBaseY", "InjPenA", "InjPenB", "InjPenC", "BOB5DefY": Value Change {
            # "Find sub-panel index"
            # "opening or closing a sub-panel"
            n176 = event-data() -> ("CtlRef"=w270:refnum<vi>)  [unwired: 1 in, 3 out]
            n177 = Search 1D Array(1D array=w269, element=w270) -> (index of element=w275:i32)  [unwired: 1 in]
            n178 = Index Array(array=w276, index=w275) -> (element=w273:refnum<vi>)
            n179 = invoke class="Bool" method="Reinit To Default"(reference=w270) -> ()  [unwired: 2 in, 3 out]
            n180 = property class="VI"(reference=w273) -> ("Front Panel.Open"=w272:bool)  [unwired: 1 in, 2 out]
            n181 = case "Panel Already Open?" shown="False" w272 {
              tunnel: w270 -> [w278 _]
              tunnel: w273 -> [_ w280]
              tunnel: [w277 refnum<vi> refnum ("vi reference")] -> w271
              frame False {
                n182 = call "OpenPanel.vi"("CtlRef"=w278) -> ("vi reference"=w277:refnum<vi>)  [unwired: 2 in]
              }
              frame True {
                n183 = call "PanelClose.vi"("vi reference"=w280) -> ()
              }
            }
            n184 = Replace Array Subset(array=w276, new element=w271, index=w275) -> (w274:refnum<vi>[])
          }
          event "Close All Panels": Value Change {
            n185 = event-data() -> ()  [unwired: 1 in, 6 out]
            n186 = case "Close Open Panels?" shown="True" "Close All Panels" {
              tunnel: w283 -> [w284 w286]
              tunnel: [w284 w285] -> w281
              frame False {
              }
              frame True {
                n187 = for "Close Open Panels" {
                  tunnel: w286 -> [w288] mode=indexing
                  tunnel: w286 -> [w287]
                  tunnel: [w287] -> w285
                  n188 = call "PanelClose.vi"("vi reference"=w288) -> ()
                }
              }
            }
          }
          event Timeout {
            # "Timeout"
            n189 = event-data() -> ()  [unwired: 1 in, 3 out]
          }
          event Panel Close? {
            n190 = event-data() -> ()  [unwired: 1 in, 4 out]
            n191 = stacked-sequence {
              tunnel: w293 -> [w298 _]
              tunnel: w292 -> [w297 _]
              tunnel: w291 -> [w296 _]
              tunnel: w290 -> [w300 _]
              frame #0 {
                # "Release DIM Services"
                n192 = for "Close Open Panels" {
                  tunnel: w300 -> [w310] mode=indexing
                  n193 = call "PanelClose.vi"("vi reference"=w310) -> ()
                }
                n194 = for "For Each Service" {
                  tunnel: w298 -> [w308] mode=indexing
                  n195 = Not A Number/Path/Refnum?(number/path/refnum=w308) -> (NaN/Path/Refnum?=w307:bool)
                  n196 = case "Not a Reference?" shown="False" w307 {
                    tunnel: w308 -> [w309 _]
                    frame False {
                      n197 = call "DimIndicators.dic_release_service.vi"("controlRef"=w309) -> ()  [unwired: 18 in, 1 out]
                    }
                    frame True {
                    }
                  }
                }
                n198 = for "For Each Service" {
                  tunnel: w297 -> [w305] mode=indexing
                  n199 = Not A Number/Path/Refnum?(number/path/refnum=w305) -> (NaN/Path/Refnum?=w304:bool)
                  n200 = case "Not a Reference?" shown="False" w304 {
                    tunnel: w305 -> [w306 _]
                    frame False {
                      n201 = call "DimIndicators.dic_release_service.vi"("controlRef"=w306) -> ()  [unwired: 18 in, 1 out]
                    }
                    frame True {
                    }
                  }
                }
                n202 = for "For Each Service" {
                  tunnel: w296 -> [w302] mode=indexing
                  n203 = Not A Number/Path/Refnum?(number/path/refnum=w302) -> (NaN/Path/Refnum?=w301:bool)
                  n204 = case "Not a Reference?" shown="False" w301 {
                    tunnel: w302 -> [w303 _]
                    frame False {
                      n205 = call "DimIndicators.dic_release_service.vi"("controlRef"=w303) -> ()  [unwired: 18 in, 1 out]
                    }
                    frame True {
                    }
                  }
                }
                n206 = control-ref of="SetFileLocation_Data"() -> (w295:refnum<vi>)
                n207 = control-ref of="Last Loaded File_Data"() -> (w299:refnum<vi>)
                n208 = call "DimIndicators.dic_release_service.vi"("controlRef"=w295) -> ()  [unwired: 18 in, 1 out]
                n209 = call "DimIndicators.dic_release_service.vi"("controlRef"=w299) -> ()  [unwired: 18 in, 1 out]
              }
              frame #1 {
                # "Close Front Panel"
                n210 = Current VI's Path() -> (path=w314:path)
                n211 = Open VI Reference(vi path=w314) -> (vi reference=w312:refnum<vi>, error out=w311:errorcluster)  [unwired: 5 in]
                n212 = property class="VI"(reference=w312, error in=w311, "Front Panel Window:Open"=FALSE) -> ()  [unwired: 2 out]
              }
            }
            n213 = event-data() -> ()  [unwired: 2 in, 1 out]
          }
        }
      }
    }
    frame #3 {
      n214 = stacked-sequence {
        tunnel: w318 -> [w320 _ _]
        tunnel: w317 -> [w324 _ _]
        tunnel: w316 -> [w321 _ _]
        tunnel: w315 -> [w322 _ _]
        frame #0 {
          # "Release DIM Services"
          n215 = control-ref of="Last Loaded File_Data"() -> (w323:refnum<vi>)
          n216 = control-ref of="SetFileLocation_Data"() -> (w319:refnum<vi>)
          n217 = call "DimIndicators.dic_release_service.vi"("controlRef"=w323) -> ()  [unwired: 18 in, 1 out]
          n218 = call "DimIndicators.dic_release_service.vi"("controlRef"=w319) -> ()  [unwired: 18 in, 1 out]
          n219 = for "For Each Service" {
            tunnel: w322 -> [w332] mode=indexing
            n220 = Not A Number/Path/Refnum?(number/path/refnum=w332) -> (NaN/Path/Refnum?=w331:bool)
            n221 = case "Not a Reference?" shown="False" w331 {
              tunnel: w332 -> [w333 _]
              frame False {
                n222 = call "DimIndicators.dic_release_service.vi"("controlRef"=w333) -> ()  [unwired: 18 in, 1 out]
              }
              frame True {
              }
            }
          }
          n223 = for "For Each Service" {
            tunnel: w321 -> [w329] mode=indexing
            n224 = Not A Number/Path/Refnum?(number/path/refnum=w329) -> (NaN/Path/Refnum?=w328:bool)
            n225 = case "Not a Reference?" shown="False" w328 {
              tunnel: w329 -> [w330 _]
              frame False {
                n226 = call "DimIndicators.dic_release_service.vi"("controlRef"=w330) -> ()  [unwired: 18 in, 1 out]
              }
              frame True {
              }
            }
          }
          n227 = for "For Each Service" {
            tunnel: w320 -> [w326] mode=indexing
            n228 = Not A Number/Path/Refnum?(number/path/refnum=w326) -> (NaN/Path/Refnum?=w325:bool)
            n229 = case "Not a Reference?" shown="False" w325 {
              tunnel: w326 -> [w327 _]
              frame False {
                n230 = call "DimIndicators.dic_release_service.vi"("controlRef"=w327) -> ()  [unwired: 18 in, 1 out]
              }
              frame True {
              }
            }
          }
          n231 = for "Close Open Panels" {
            tunnel: w324 -> [w334] mode=indexing
            n232 = call "PanelClose.vi"("vi reference"=w334) -> ()
          }
        }
        frame #1 {
          # "Close Front Panel"
          n233 = Current VI's Path() -> (path=w335:path)
          n234 = Open VI Reference(vi path=w335) -> (vi reference=w337:refnum<vi>, error out=w338:errorcluster)  [unwired: 5 in]
          n235 = property class="VI"(reference=w337, error in=w338, "Front Panel Window:Open"=FALSE) -> ()  [unwired: 2 out]
        }
        frame #2 {
          # "Stop Panel"
          n236 = Stop(stop? (T)=TRUE) -> ()
        }
      }
    }
  }
  n237 = call "LVDimInterface.dim_operate.vi"("DNSNode"="lebit-balcony" ("DNS node")) -> ()  [unwired: 19 in]
